vi "Read Base URL.vi"(8 "error in (no error)":errorcluster, 11 "REST Interface in":refnum<class "REST Interface.lvclass">) -> (0 "error out":errorcluster, 2 "Base URL":string, 3 "REST Interface out":refnum<class "REST Interface.lvclass">)   [LabVIEW 2018, in "REST Interface.lvlib" / "REST Interface.lvclass"]
uses:
  REST Interface.lvclass
  REST Interface.lvclass/REST Interface.ctl
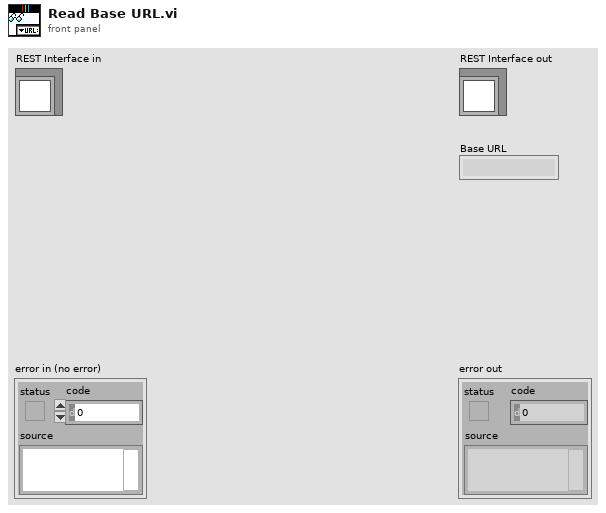
[diagram p1: front panel]
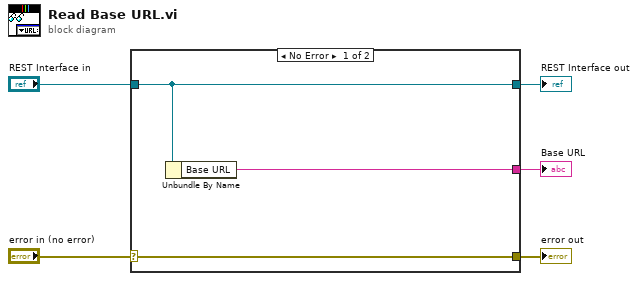
[diagram p0: block diagram]
diagram:
  n1 = case shown="No Error" "error in (no error)" {
    selector: "error in (no error)" -> [w8 w9]
    tunnel: [w8 w9] -> w4
    tunnel: [w7 w10] -> w2
    tunnel: "REST Interface in" -> [w7 w10]
    tunnel: [w6 _] -> w1
    frame No Error {
      n2 = Unbundle By Name(w7) -> ("Base URL"=w6:string)
    }
    frame Error {
    }
  }
  "error out" <- w4
  "REST Interface out" <- w2
  "Base URL" <- w1
